vi "new  process file - Copy.vi"() -> ()   [LabVIEW 2018]
panel:
  in  "SET":bool
  in  "n of bilayer":dbl
  in  "process name":string
  out "count":dbl
  out "multiple":string
  out "single":string
  in  "SEARCH":bool
  in  "EXIT":bool
  in  "SAVE":bool
  in  "DELETE":bool
  in  "ADD":bool
  # "Process Name"
  # "Recipe Name"
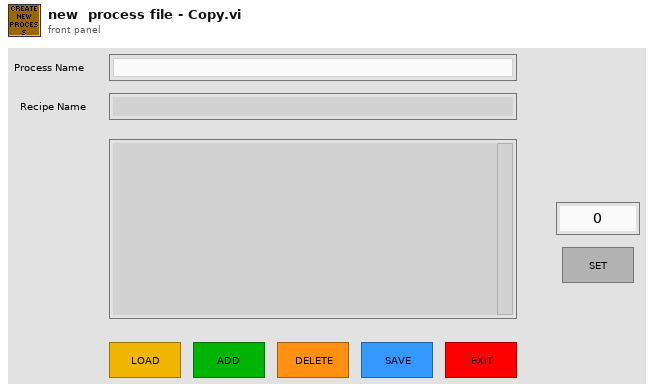
[diagram p1: front panel]
types:
  T1 = enum16{"open", "replace", "create", "open or create", "replace or create", "replace or create with confirmation"}
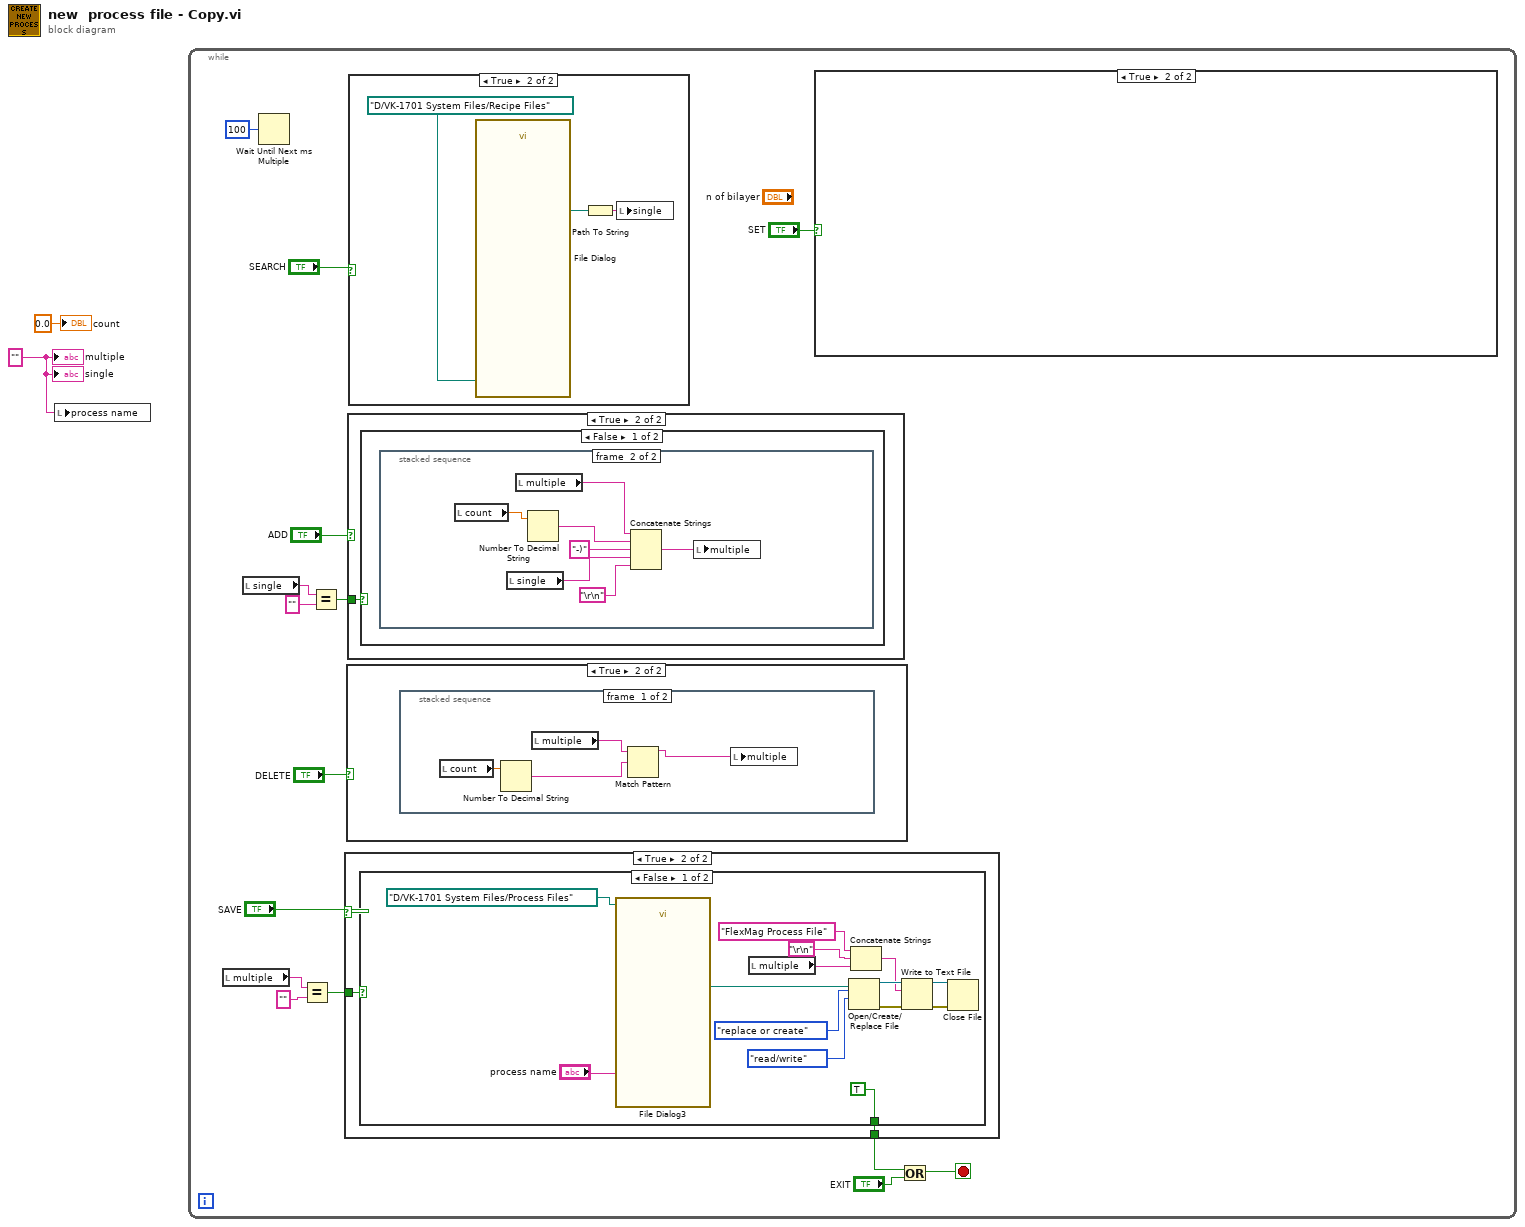
[diagram p0: block diagram]
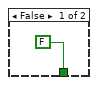
[diagram p3: hidden frame]
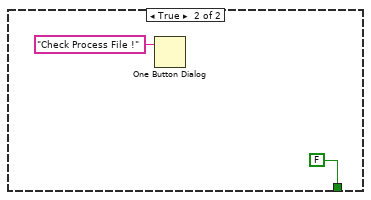
[diagram p4: hidden frame]
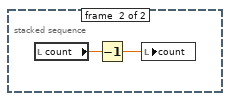
[diagram p6: hidden frame]
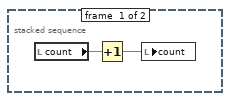
[diagram p8: hidden frame]
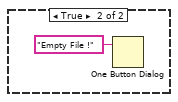
[diagram p9: hidden frame]
diagram:
  w1 = "" ("multiple")
  n1 = local write "process name"(w1) -> ()
  n2 = while {
    stop <- w4 stop-if-true
    n3 = local read "multiple"() -> (w8:string)
    n4 = local read "single"() -> (w15:string)
    n5 = Wait Until Next ms Multiple(millisecond multiple=u32 100) -> ()  [unwired: 1 out]
    n6 = Equal?(x=w8, y="") -> (x = y?=w7:bool)
    n7 = Equal?(x=w15, y="") -> (x = y?=w13:bool)
    n8 = case shown="True" "SAVE" {
      tunnel: w7 -> [_ w20]
      tunnel: [FALSE w19] -> w5
      frame False {
      }
      frame True {
        n9 = case shown="False" w20 {
          tunnel: [TRUE FALSE] -> w19
          frame False {
            n10 = call "File Dialog3"("start path"=path "D:/VK-1701 System Files/Process Files", "default name"="process name") -> ("selected path"=w30:path)  [unwired: 10 in, 3 out]
            n11 = local read "multiple"() -> (w23:string)
            n12 = Open/Create/Replace File(file path (use dialog)=w30, operation (0:open)=T1."replace or create", access (0:read/write)=enum16{"read/write", "read-only", "write-only"}."read/write") -> (refnum out=w27:refnum<file>, error out=w26:errorcluster)  [unwired: 3 in, 1 out]
            n13 = Concatenate Strings("FlexMag Process File" ("y"), "\r\n", w23) -> (w24:string)
            n14 = Write to Text File(file (use dialog)=w27, text=w24, error in=w26) -> (refnum out=w29:refnum<file>, error out=w28:errorcluster)  [unwired: 1 in, 1 out]
            n15 = Close File(refnum=w29, error in=w28) -> ()  [unwired: 2 out]
          }
          frame True {
            n16 = One Button Dialog(message="Check Process File !") -> ()  [unwired: 1 in, 1 out]
          }
        }
      }
    }
    n17 = case shown="True" "DELETE" {
      frame False {
      }
      frame True {
        n18 = stacked-sequence {
          frame #0 {
            n19 = local read "count"() -> (w40:dbl)
            n20 = Number To Decimal String(number=w40) -> (decimal integer string=w38:string)  [unwired: 1 in]
            n21 = local read "multiple"() -> (w39:string)
            n22 = Match Pattern(string=w39, regular expression=w38) -> (before substring=w37:string)  [unwired: 1 in, 3 out]
            n23 = local write "multiple"(w37) -> ()
          }
          frame #1 {
            n24 = local read "count"() -> (w42:dbl)
            n25 = Decrement(x=w42) -> (x-1=w41:dbl)
            n26 = local write "count"(w41) -> ()
          }
        }
      }
    }
    n27 = case shown="True" "ADD" {
      tunnel: w13 -> [_ w43]
      frame False {
      }
      frame True {
        n28 = case shown="False" w43 {
          frame False {
            n29 = stacked-sequence {
              frame #0 {
                n30 = local read "count"() -> (w44:dbl)
                n31 = Increment(x=w44) -> (x+1=w45:dbl)
                n32 = local write "count"(w45) -> ()
              }
              frame #1 {
                n33 = local read "count"() -> (w52:dbl)
                n34 = local read "single"() -> (w49:string)
                n35 = local read "multiple"() -> (w47:string)
                n36 = Number To Decimal String(number=w52) -> (decimal integer string=w51:string)  [unwired: 1 in]
                n37 = Concatenate Strings(w47, w51, "-)" ("string"), w49, "\r\n") -> (w48:string)
                n38 = local write "multiple"(w48) -> ()
              }
            }
          }
          frame True {
            n39 = One Button Dialog(message="Empty File !") -> ()  [unwired: 1 in, 1 out]
          }
        }
      }
    }
    n40 = case shown="True" "SEARCH" {
      frame False {
      }
      frame True {
        n41 = call "File Dialog"("start path"=path "D:/VK-1701 System Files/Recipe Files") -> ("selected path"=w55:path)  [unwired: 11 in, 3 out]
        n42 = Path To String(path=w55) -> (string=w54:string)
        n43 = local write "single"(w54) -> ()
      }
    }
    n44 = case shown="True" "SET" {
      frame False {
      }
      frame True {
      }
    }
    n45 = Or(x=w5, y="EXIT") -> (x .or. y?=w4:bool)
  }
  "multiple" <- w1
  "count" <- 0.0 ("count")
  "single" <- w1
